vi "MakeAndSendDataValuesOMFJSON.vi"(0 "client handle":T2, 1 "OMF Ingress URL":string, 5 "OMF Container ID":string, 7 "OMF Dynamic Type Property Names and Formats":T1(array[cluster])=[{"Dynamic Property Name"="X acceleration", "Dynamic Property Format"=enum."string"}, {"Dynamic Property Name"="Y acceleration", "Dynamic Property Format"=enum."string"}, {"Dynamic Property Name"="Z acceleration", "Dynamic Property Format"=enum."string"}], 9 "Array of Values":string[](array[string]), 11 "error in (no error)":errorcluster) -> (6 "Response headers for continuous OMF data messages":string, 8 "Reponse body for continuous OMF data messages":string, 15 "error out":errorcluster)   [LabVIEW 2014]
uses:
  <vilib>/httpClient/ClientHandle.ctl
  <vilib>/httpClient/LabVIEWHTTPClient.lvlib
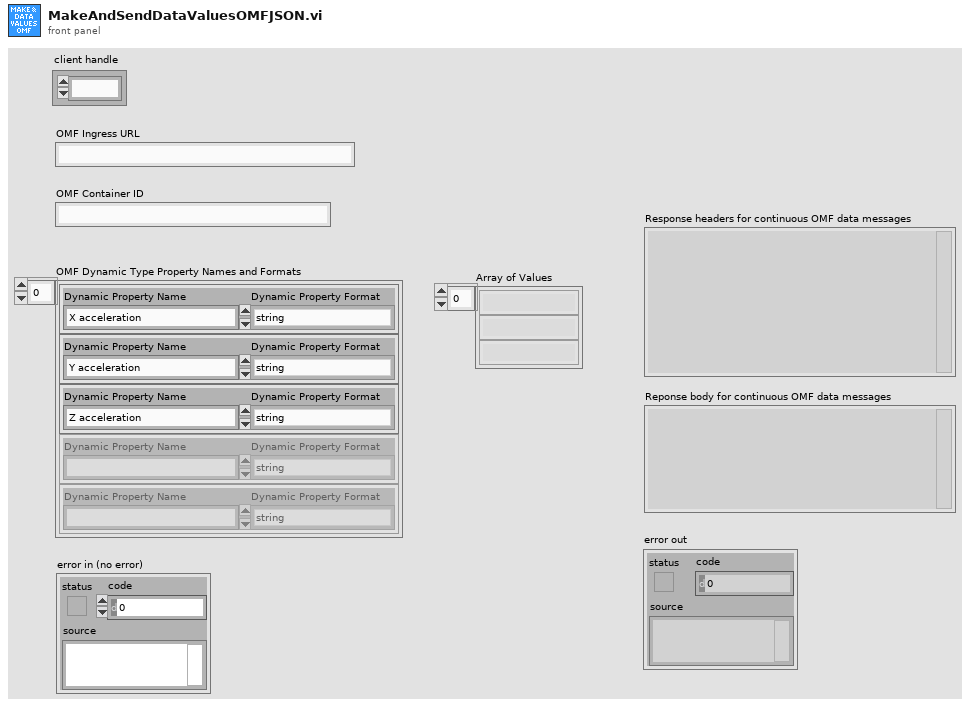
[diagram p1: front panel]
types:
  T1 = cluster{"Dynamic Property Name":string, "Dynamic Property Format":enum16{"string", "number"}}[]
  T2 = typedef "LabVIEWHTTPClient.lvlib/ClientHandle.ctl" = refnum<k1>
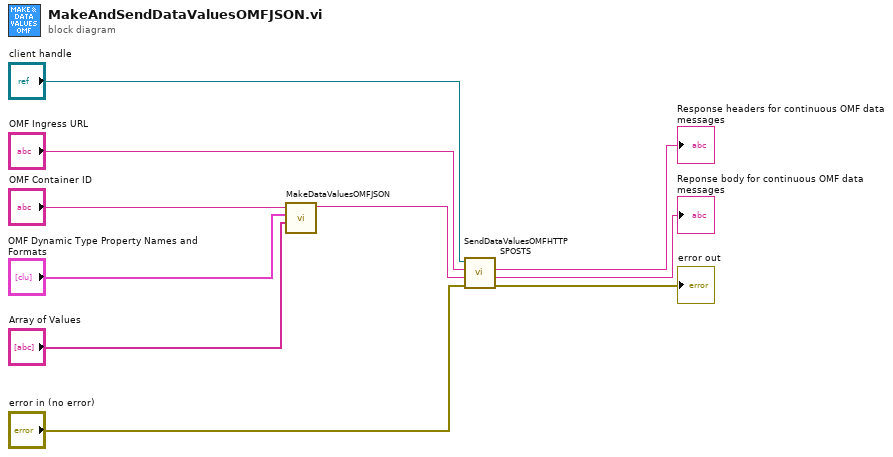
[diagram p0: block diagram]
diagram:
  n1 = call "MakeDataValuesOMFJSON.vi"("Array of Values"="Array of Values", "OMF Dynamic Type Property Names and Formats"="OMF Dynamic Type Property Names and Formats", "OMF Container ID"="OMF Container ID") -> ("OMF Data Values JSON"=w8:string)  [unwired: 8 in]
  n2 = call "SendDataValuesOMFHTTPSPOSTS.vi"("error in (no error)"="error in (no error)", "OMF Data Values JSON"=w8, "OMF Ingress URL"="OMF Ingress URL", "client handle"="client handle") -> ("error out"=→"error out":errorcluster, "Reponse body for continuous OMF data messages"=→"Reponse body for continuous OMF data messages":string, "Response headers for continuous OMF data messages"=→"Response headers for continuous OMF data messages":string)  [unwired: 3 in]
